vi "Append Control Image to Report.vi"(0 "report in":refnum<class "ooCalc.lvclass">, 1 "alignment (default)":T2, 2 "image file type (.jpg)":enum16{".jpg", ".png"}(ring), 5 "image depth":T1=2 items=["B&W", "4 bits", "8 bits", "24 bits"], 7 "ctrl reference":refnum<vi>, 9 "description":string, 11 "error in (no error)":errorcluster, 12 "MS Office parameters":T3) -> (4 "report out":refnum<class "ooCalc.lvclass">, 8 "start out (Word)":i32, 10 "end out (Word)":i32, 15 "error out":errorcluster)   [LabVIEW 2009, in "ooCalc.lvclass"]
doc: "Creates an image of the front panel object specified in <B>ctrl reference</B> and appends it to a report."
uses:
  ooCalc.lvclass
  <vilib>/Utility/NIReport.llb/HTML Report Image Alignment.ctl
  <vilib>/Utility/NIReport.llb/image depth.ctl
  <vilib>/Utility/NIReport.llb/NI_ReportGenerationCore.lvlib
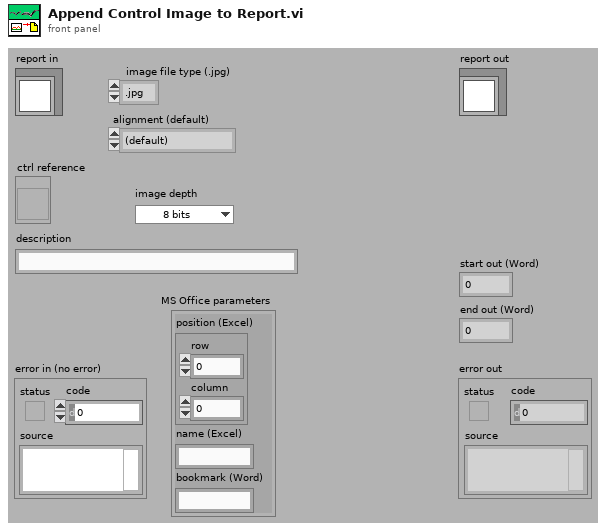
[diagram p1: front panel]
types:
  T1 = typedef "NI_ReportGenerationCore.lvlib/image depth.ctl" = u16
  T2 = typedef "NI_ReportGenerationCore.lvlib/HTML Report Image Alignment.ctl" = enum16{"(default)", "LEFT", "RIGHT", "TOP", "TEXTTOP", "MIDDLE", "ABSMIDDLE", "BASELINE", "BOTTOM", "ABSBOTTOM"}
  T3 = cluster{"position (Excel)":cluster{"row":i32, "column":i32}, "name (Excel)":string, "bookmark (Word)":string}
  T4 = typedef "imagedata.ctl" = cluster{"image type":i32, "image depth":i32, "image":u8[], "mask":u8[], "colors":u32[], "Rectangle":cluster{"left":i16, "top":i16, "right":i16, "bottom":i16}}
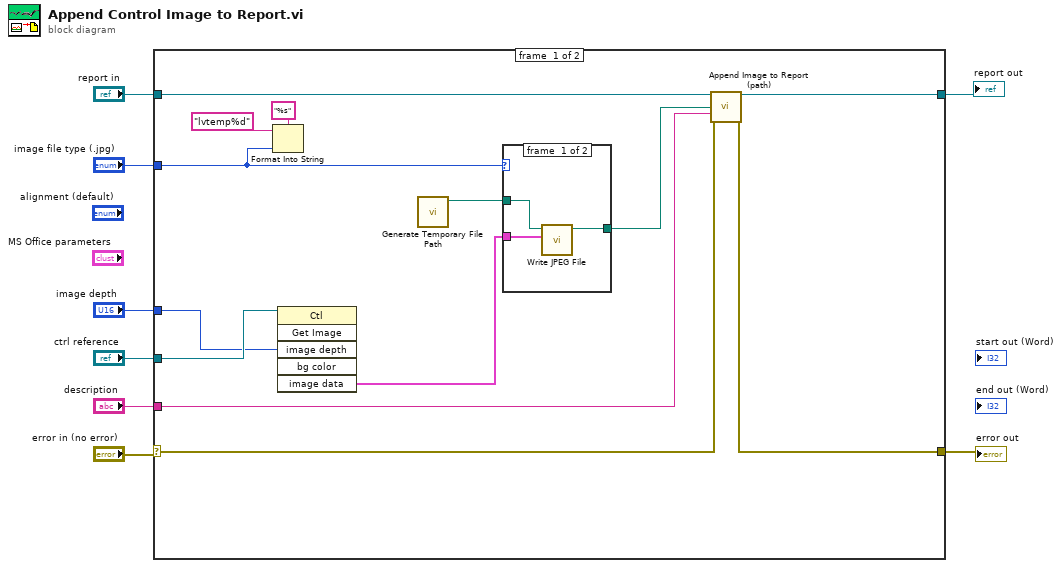
[diagram p0: block diagram]
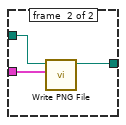
[diagram p2: hidden frame]
diagram:
  n1 = case shown="No Error" "error in (no error)" {
    selector: "error in (no error)" -> [w11 w28]
    tunnel: [w10 w28] -> w7
    tunnel: "report in" -> [w21 w29]
    tunnel: [w20 w29] -> w5
    tunnel: "description" -> [w19 _]
    tunnel: "ctrl reference" -> [w18 _]
    tunnel: "image depth" -> [w17 _]
    tunnel: "image file type (.jpg)" -> [w14 _]
    frame #0 {
      n2 = Format Into String(format string="%s", initial string="lvtemp%d" ("pattern (lvtemp%d.tmp)"), w14) -> ()  [unwired: 1 in, 2 out]
      n3 = invoke class="Ctl" method="Get Image"(reference=w18, "image depth"=w17) -> ("image data"=w16:T4)  [unwired: 4 in, 5 out]
      n4 = call <vilib>:"Generate Temporary File Path.vi"() -> ("Unique Temporary File Path"=w9:path)  [unwired: 10 in, 1 out]
      n5 = case shown="\".png\"" w14 {
        tunnel: w16 -> [w24 w27]
        tunnel: w9 -> [w23 w26]
        tunnel: [w22 w25] -> w15
        frame #0 {
          n6 = call <vilib>:"Write JPEG File.vi"("image data"=w24, "path to JPEG file"=w23) -> ("path"=w22:path)  [unwired: 8 in, 1 out]
        }
        frame #1 {
          n7 = call <vilib>:"Write PNG File.vi"("image data"=w27, "path to PNG file"=w26) -> ("path"=w25:path)  [unwired: 8 in, 1 out]
        }
      }
      n8 = call-dynamic "Append Image to Report (path).vi"("report in"=w21, "path or URL of image"=w15, "caption or alternative string"=w19, "error in (no error)"=w11) -> ("report out"=w20:refnum<class "ooCalc.lvclass">, "error out"=w10:errorcluster)  [unwired: 8 in, 2 out]
    }
    frame #1 {
    }
  }
  "error out" <- w7
  "report out" <- w5
